vi "Ramp Vector I32, New.vi"(1 "step (1)":i32=1, 2 "nelem":i32=5, 3 "start (0)":i32) -> (0 "ramp":i32[](array[numeric]))   [LabVIEW 2010]
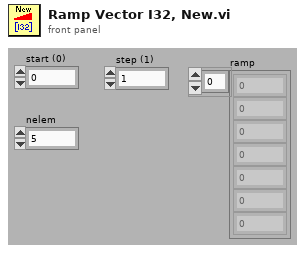
[diagram p1: front panel]
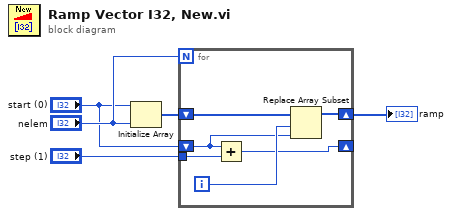
[diagram p0: block diagram]
diagram:
  n1 = Initialize Array("start (0)", "nelem") -> (w5:i32[])
  n2 = for {
    N: "nelem" -> [_]
    shift-right: [w11] -> w4
    shift-left: w5 -> [w10]
    shift-right: [w7] -> _
    shift-left: "start (0)" -> [w6]
    tunnel: "step (1)" -> [w8]
    i -> [w9]
    n3 = Add(x=w6, y=w8) -> (x+y=w7:i32)
    n4 = Replace Array Subset(array=w10, new element=w6, index=w9) -> (w11:i32[])
  }
  "ramp" <- w4
